vi "Stop all movement.vi"(8 "error in (no error)":errorcluster, 11 "XYZ Stage Control in":refnum<class "XYZ Stage Control.lvclass">) -> (0 "error out":errorcluster, 2 "XYZ Position Set":T1={"Speed"=0, "Z Limit (um+/-)"=0.0, "Axes"="All", "XYZ Coordinates"={"X"=0.0, "Y"=0.0, "Z"=0.0}} {"XYZ Coordinates"."Z" format="Z= %#_g"; "XYZ Coordinates"."Y" format="Y= %#_g"; "XYZ Coordinates"."X" format="X= %#_g"; "Z Limit (um+/-)" format="Z Limit = %.0f"; "Speed" format="Speed= %.0f"}, 3 "XYZ Stage Control out":refnum<class "XYZ Stage Control.lvclass">)   [LabVIEW 2020, in "TranslationStageClassStructure.lvlib" / "XYZ Stage Control.lvclass"]
uses:
  XYZ Stage Control.lvclass
  typedefs/XYZ_position_input.ctl
  typedefs/XYZ axes.ctl
  Typedefs/XYZ_coordinates.ctl
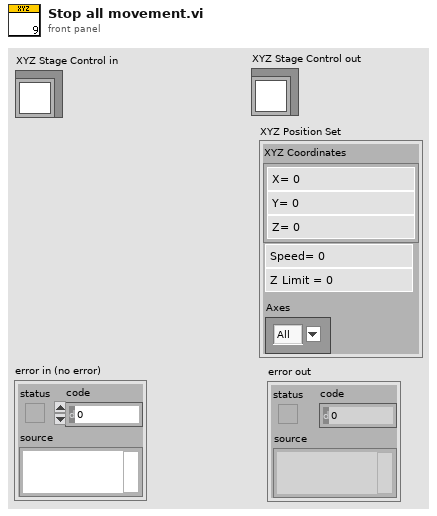
[diagram p1: front panel]
types:
  T1 = typedef "XYZ_position_input.ctl" = cluster{"Speed":i32, "Z Limit (um+/-)":sgl, "Axes":T2, "XYZ Coordinates":T3}
  T2 = typedef "XYZ axes.ctl" = string
  T3 = typedef "XYZ_coordinates.ctl" = cluster{"X":sgl, "Y":sgl, "Z":sgl}
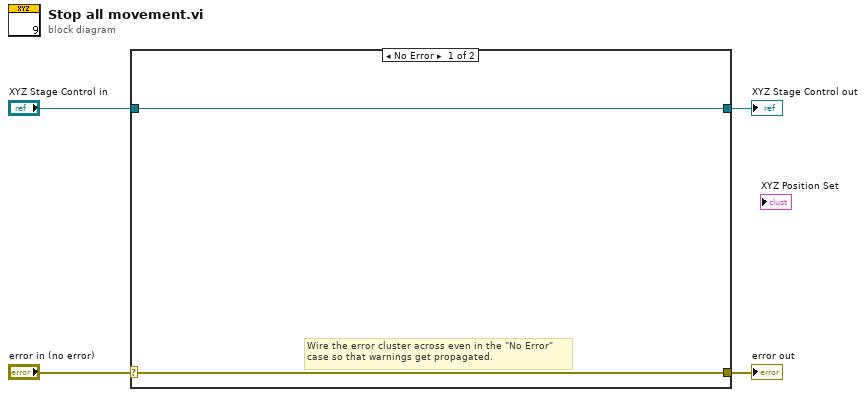
[diagram p0: block diagram]
diagram:
  n1 = case shown="No Error" "error in (no error)" {
    selector: "error in (no error)" -> [w5 w8]
    tunnel: [w5 w8] -> w3
    tunnel: [w6 w7] -> w1
    tunnel: "XYZ Stage Control in" -> [w6 w7]
    frame No Error {
      # "Wire the error cluster across even in the \"No Error\"\ncase so that warnings get propagated."
    }
    frame Error {
    }
  }
  "error out" <- w3
  "XYZ Stage Control out" <- w1
